vi "Read Git Info.vi"(6 "Short Hash Length (7)":i32=7, 8 "error in (no error)":errorcluster, 11 "System Config Module in":refnum<class "System Config Module.lvclass">) -> (0 "error out":errorcluster, 1 "Commit":string, 2 "Latest Tag":string, 3 "System Config Module out":refnum<class "System Config Module.lvclass">, 4 "Short Hash":string, 5 "Branch":string)   [LabVIEW 2020, in "Volatus.lvlib" / "System Config Module.lvclass"]
uses:
  System Config Module.lvclass
  <vilib>/Hampel Software Engineering/Git API/Git API/GIT-api.lvclass/GIT-api.ctl
  System Config Module.lvclass/System Config Module.ctl
  <vilib>/Hampel Software Engineering/Git API/Git API/GIT-api.lvclass
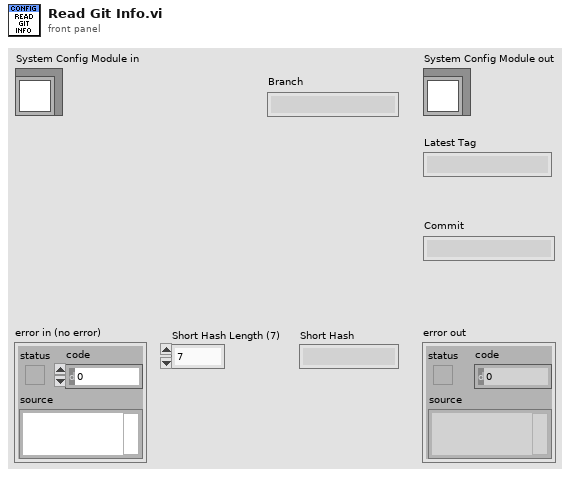
[diagram p1: front panel]
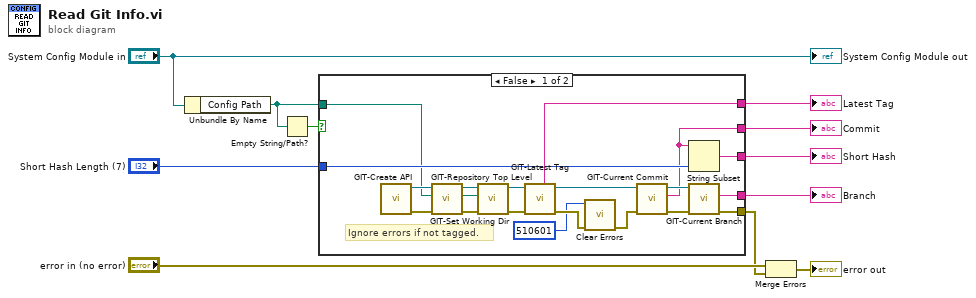
[diagram p0: block diagram]
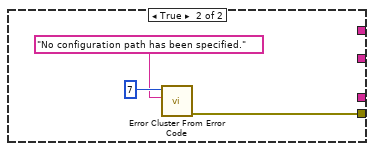
[diagram p2: hidden frame]
diagram:
  n1 = Unbundle By Name("System Config Module in") -> ("Config Path"=w2:path)
  n2 = Empty String/Path?(string/path=w2) -> (empty?=w1:bool)
  n3 = case shown="False" w1 {
    tunnel: [w24 _] -> w9
    tunnel: [w20 w34] -> w7
    tunnel: "Short Hash Length (7)" -> [w16 _]
    tunnel: [w15 _] -> w5
    tunnel: [w14 _] -> w4
    tunnel: [w13 _] -> w3
    tunnel: w2 -> [w12 _]
    frame False {
      # "Ignore errors if not tagged."
      n4 = call <vilib>:"GIT-Create API.vi"() -> ("error out"=w30:errorcluster, "git-api out"=w31:refnum<class "GIT-api.lvclass">)  [unwired: 10 in]
      n5 = call <vilib>:"GIT-Repository Top Level.vi"("error in"=w30, "Current Path"=w12, "git-api in"=w31) -> ("error out"=w27:errorcluster, "Repo Top Level Path"=w28:path, "git-api out"=w29:refnum<class "GIT-api.lvclass">)  [unwired: 6 in]
      n6 = call <vilib>:"GIT-Set Working Dir.vi"("error in"=w27, "Working Directory"=w28, "git-api in"=w29) -> ("error out"=w26:errorcluster, "git-api out"=w25:refnum<class "GIT-api.lvclass">)  [unwired: 7 in]
      n7 = call <vilib>:"GIT-Latest Tag.vi"("error in"=w26, "git-api in"=w25) -> ("error out"=w19:errorcluster, "git-api out"=w23:refnum<class "GIT-api.lvclass">, "Latest Tag"=w24:string)  [unwired: 6 in, 1 out]
      n8 = call <vilib>:"Clear Errors.vi"("error in (no error)"=w19, "specific error code to clear (0: all)"=510601) -> ("error out"=w18:errorcluster)  [unwired: 4 in, 1 out]
      n9 = call <vilib>:"GIT-Current Commit.vi"("error in"=w18, "git-api in"=w23) -> ("error out"=w21:errorcluster, "current commit"=w13:string, "git-api out"=w22:refnum<class "GIT-api.lvclass">)  [unwired: 7 in]
      n10 = String Subset(string=w13, length (rest)=w16) -> (substring=w15:string)  [unwired: 1 in]
      n11 = call <vilib>:"GIT-Current Branch.vi"("error in"=w21, "git-api in"=w22) -> ("error out"=w20:errorcluster, "current branch"=w14:string)  [unwired: 6 in, 2 out]
    }
    frame True {
      n12 = call <vilib>:"Error Cluster From Error Code.vi"("error message (\"\")"="No configuration path has been specified." ("error message (\"\")"), "error code (0)"=7) -> ("error out"=w34:errorcluster)  [unwired: 7 in]
    }
  }
  "Latest Tag" <- w9
  "Short Hash" <- w5
  "Commit" <- w3
  "Branch" <- w4
  n13 = Merge Errors("error in (no error)", w7) -> (→"error out":errorcluster)
  "System Config Module out" <- "System Config Module in"
